vi "get dns name from windows.vi"() -> (0 "ToString":string)   [LabVIEW 2017]
uses:
  System.Management
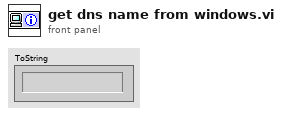
[diagram p1: front panel]
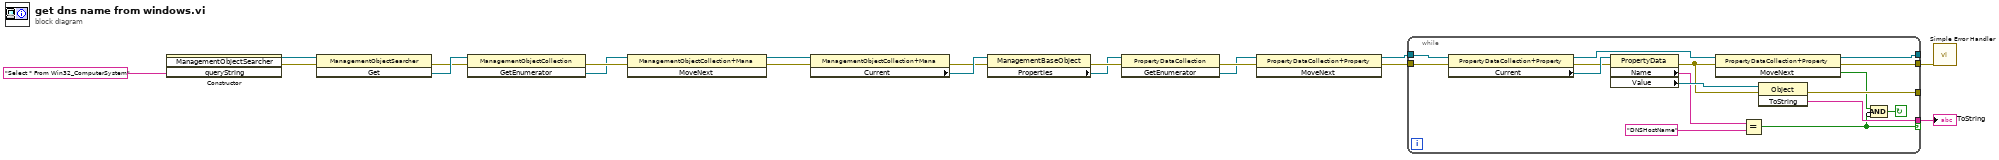
[diagram p0: block diagram]
diagram:
  n1 = constructor class="ManagementObjectSearcher"("queryString"="Select * From Win32_ComputerSystem" ("query")) -> (reference out=w15:refnum<k24>, error out=w14:errorcluster)  [unwired: 3 in, 2 out]
  n2 = invoke class="ManagementObjectSearcher" method="Get"(reference=w15, error in=w14) -> (error out=w16:errorcluster, "Get"=w17:refnum<k24>)  [unwired: 1 in, 1 out]
  n3 = invoke class="ManagementObjectCollection" method="GetEnumerator"(reference=w17, error in=w16) -> (error out=w19:errorcluster, "GetEnumerator"=w18:refnum<k24>)  [unwired: 1 in, 1 out]
  n4 = invoke class="ManagementObjectCollection+Mana" method="MoveNext"(reference=w18, error in=w19) -> (reference out=w12:refnum<k24>, error out=w11:errorcluster)  [unwired: 1 in, 1 out]
  n5 = property class="ManagementObjectCollection+Mana"(reference=w12, error in=w11) -> (error out=w3:errorcluster, "Current"=w4:refnum<k24>)  [unwired: 1 out]
  n6 = property class="ManagementBaseObject"(reference=w4, error in=w3) -> (error out=w8:errorcluster, "Properties"=w5:refnum<k24>)  [unwired: 1 out]
  n7 = invoke class="PropertyDataCollection" method="GetEnumerator"(reference=w5, error in=w8) -> (error out=w9:errorcluster, "GetEnumerator"=w6:refnum<k24>)  [unwired: 1 in, 1 out]
  n8 = invoke class="PropertyDataCollection+Property" method="MoveNext"(reference=w6, error in=w9) -> (reference out=w7:refnum<k24>, error out=w10:errorcluster)  [unwired: 1 in, 1 out]
  n9 = while {
    tunnel: w7 -> [w35]
    tunnel: w10 -> [w33]
    tunnel: [w30] -> w2
    tunnel: [w29] -> _
    tunnel: [w26] -> _
    tunnel: [w23] -> w1 if=w21
    stop <- w20 continue-if-true
    n10 = property class="PropertyDataCollection+Property"(reference=w35, error in=w33) -> (reference out=w32:refnum<k24>, error out=w31:errorcluster, "Current"=w34:refnum<k24>)
    n11 = property class="PropertyData"(reference=w34, error in=w31) -> (error out=w27:errorcluster, "Name"=w25:string, "Value"=w28:refnum<k24>)  [unwired: 1 out]
    n12 = invoke class="PropertyDataCollection+Property" method="MoveNext"(reference=w32, error in=w27) -> (reference out=w29:refnum<k24>, error out=w30:errorcluster, "MoveNext"=w22:bool)  [unwired: 1 in]
    n13 = Equal?(x=w25, y="DNSHostName") -> (x = y?=w21:bool)
    n14 = invoke class="Object" method="ToString"(reference=w28, error in=w27) -> (error out=w26:errorcluster, "ToString"=w23:string)  [unwired: 1 in, 1 out]
    n15 = Compound Arithmetic op=AND(w22, invert w21) -> (w20:bool)
  }
  "ToString" <- w1
  n16 = call <vilib>:"Simple Error Handler.vi"("error in (no error)"=w2) -> ()  [unwired: 4 in, 5 out]
